vi "Save Learning Coeff (SubVI).vi"(10 "initialized array":dbl[](array[numeric]), 11 "Boolean":bool) -> ()   [LabVIEW 2025]
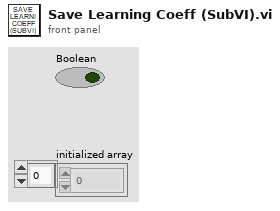
[diagram p1: front panel]
types:
  T1 = enum16{"open", "replace", "create", "open or create", "replace or create", "replace or create with confirmation"}
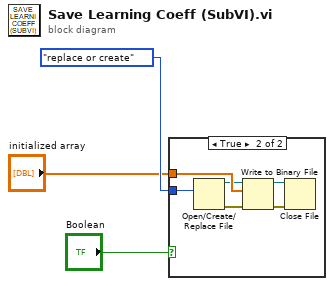
[diagram p0: block diagram]
diagram:
  n1 = case shown="True" "Boolean" {
    tunnel: "initialized array" -> [_ w9]
    tunnel: T1."replace or create" ("operation (0:open)") -> [_ w4]
    frame False {
    }
    frame True {
      n2 = Open/Create/Replace File(operation (0:open)=w4) -> (refnum out=w5:refnum<file>, error out=w6:errorcluster)  [unwired: 5 in, 1 out]
      n3 = Write to Binary File(file (use dialog)=w5, data=w9, error in=w6) -> (refnum out=w7:refnum<file>, error out=w8:errorcluster)  [unwired: 3 in, 1 out]
      n4 = Close File(refnum=w7, error in=w8) -> ()  [unwired: 2 out]
    }
  }
